vi "Enable Limits.vi"(8 "error in (no error)":errorcluster, 9 "Enable Voltage Limit (T: Enable)":bool=TRUE, 10 "Enable Current Limit (T: Enable)":bool=TRUE, 11 "VISA resource name":refnum<visa-resource-name>) -> (0 "error out":errorcluster, 3 "VISA resource name out":refnum<visa-resource-name>)   [LabVIEW 2023]
doc: "Enables or disables current and voltage limits that prevent the protection limits from being reached. This limits the current and voltage at 95% of the overcurrent protection (OCP) and overvoltage protection (OVP) respectivly. This prevents the output turning off and an alarm being produced."
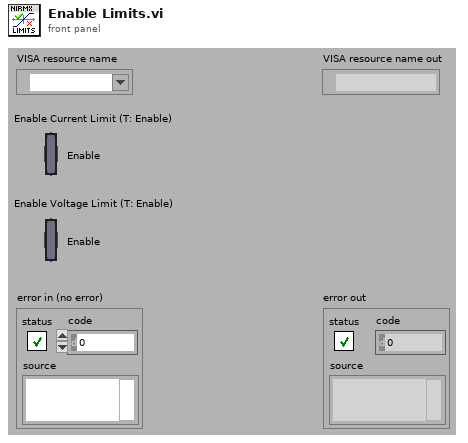
[diagram p1: front panel]
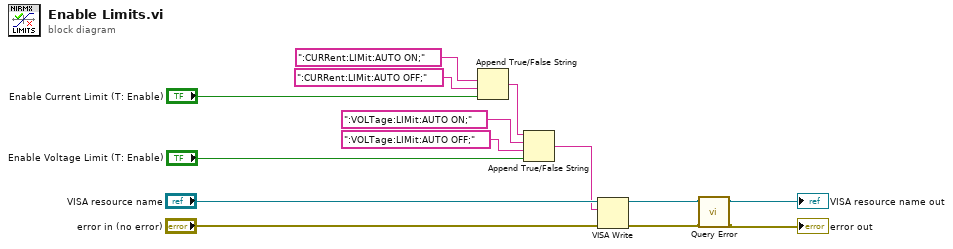
[diagram p0: block diagram]
diagram:
  n1 = Append True/False String(1:"Enable Current Limit (T: Enable)", 2:":CURRent:LIMit:AUTO OFF;", 3:":CURRent:LIMit:AUTO ON;") -> (0:w10:string)  [unwired: 1 in]
  n2 = Append True/False String(1:"Enable Voltage Limit (T: Enable)", 2:":VOLTage:LIMit:AUTO OFF;", 3:":VOLTage:LIMit:AUTO ON;", 4:w10) -> (0:w5:string)
  n3 = VISA Write(VISA resource name="VISA resource name", write buffer=w5, error in (no error)="error in (no error)") -> (VISA resource name out=w2:refnum<visa-resource-name>, error out=w1:errorcluster)  [unwired: 1 out]
  n4 = call "Query Error.vi"("error in (no error)"=w1, "VISA resource name"=w2) -> ("error out"=→"error out":errorcluster, "VISA resource name out"=→"VISA resource name out":refnum<visa-resource-name>)  [unwired: 6 in, 2 out]
